vi "stop.vi"(3 "error in (no error)":errorcluster, 4 "stop":bool, 5 "HamegHMPSupply in":refnum<class "HamegHMPSupply.lvclass">) -> (0 "error out":errorcluster, 1 "Stopped":bool, 2 "HamegHMPSupply out":refnum<class "HamegHMPSupply.lvclass">)   [LabVIEW 2009, in "Hardware.lvlib" / "Channels.lvlib" / "HamegHMPSupply.lvclass"]
doc: "Abstract Method.\n\nStops the analog output. This vi indicates of the analog output has stopped, and can be used to actively stop the output."
uses:
  HamegHMPSupply.lvclass
  AnalogOutput.lvclass
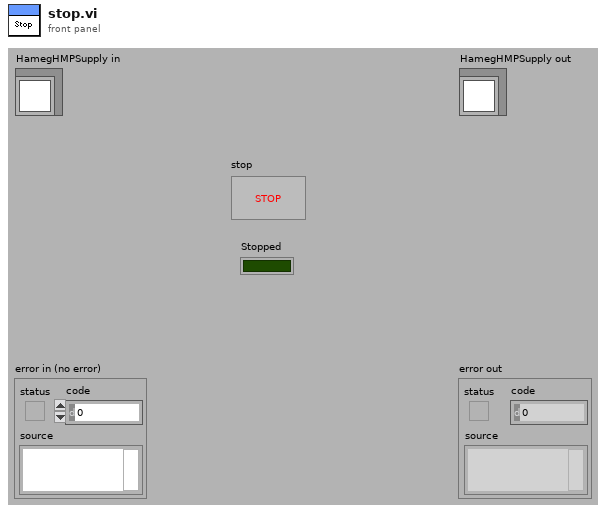
[diagram p1: front panel]
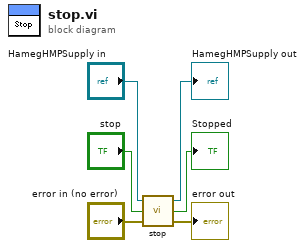
[diagram p0: block diagram]
diagram:
  n1 = call-parent "stop.vi"("error in (no error)"="error in (no error)", "stop"="stop", "AnalogOutput in"="HamegHMPSupply in") -> ("error out"=→"error out":errorcluster, "Stopped"=→"Stopped":bool, "AnalogOutput out"=→"HamegHMPSupply out":refnum<class "HamegHMPSupply.lvclass">)
